vi "Create Engine.vi"(5 "FIFO Debug Flags":refnum<class "Debug Flags FIFO.lvclass">, 7 "fifo/queue depths (10)":u32=10, 8 "error in (no error)":errorcluster, 10 "error size (512 B)":T1=enum."512-byte", 11 "Interface type":refnum<class "Engine Interface.lvclass">) -> (0 "error out":errorcluster, 3 "Interface":refnum<class "Engine Interface.lvclass">)   [LabVIEW 2017, in "Data Sharing Framework Engine.lvlib" / "Engine Interface.lvclass"]
uses:
  Engine Interface.lvclass
  Error Queue Sizes.ctl
  Debug/Debug Flags FIFO/Debug Flags FIFO.lvclass
  Engine Interface.lvclass/Engine Interface.ctl
  Create 16B RT FIFO.vi
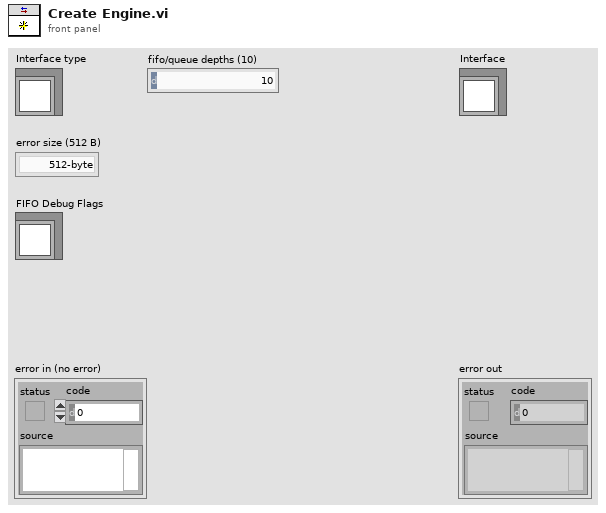
[diagram p1: front panel]
types:
  T1 = typedef "Data Sharing Framework Engine.lvlib/Engine Interface.lvclass/Error Queue Sizes.ctl" = enum16{"256-byte", "512-byte", "1024-byte"}
  T2 = typedef "Data Sharing Framework Engine.lvlib/Engine Interface.lvclass/16B RT FIFO Reference.ctl" = refnum<k33>
  T3 = typedef "Data Sharing Framework Engine.lvlib/Engine Interface.lvclass/Error Queue Ref.ctl" = refnum<queue>
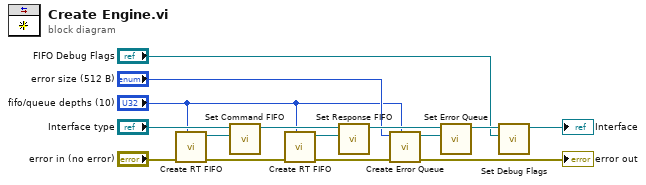
[diagram p0: block diagram]
diagram:
  n1 = call-poly "Create RT FIFO.vi"("size (10)"="fifo/queue depths (10)", "error in (no error)"="error in (no error)") -> ("error out"=w10:errorcluster, "RT FIFO"=w14:T2)  [unwired: 8 in]
  n2 = call "Set Command FIFO.vi"("Command FIFO"=w14, "Interface in"="Interface type") -> ("Interface out"=w11:refnum<class "Engine Interface.lvclass">)  [unwired: 9 in]
  n3 = call-poly "Create RT FIFO.vi"("size (10)"="fifo/queue depths (10)", "error in (no error)"=w10) -> ("error out"=w8:errorcluster, "RT FIFO"=w13:T2)  [unwired: 8 in]
  n4 = call "Set Response FIFO.vi"("Response FIFO"=w13, "Interface in"=w11) -> ("Interface out"=w9:refnum<class "Engine Interface.lvclass">)  [unwired: 9 in]
  n5 = call "Create Error Queue.vi"("max queue size (10)"="fifo/queue depths (10)", "error in (no error)"=w8, "error size"="error size (512 B)") -> ("error out"=→"error out":errorcluster, "Error Queue"=w7:T3)  [unwired: 7 in]
  n6 = call "Set Error Queue.vi"("Error Queue"=w7, "Interface in"=w9) -> ("Interface out"=w4:refnum<class "Engine Interface.lvclass">)  [unwired: 9 in]
  n7 = call "Set Debug Flags.vi"("FIFO Debug Flags"="FIFO Debug Flags", "Interface in"=w4) -> ("Interface out"=→"Interface":refnum<class "Engine Interface.lvclass">)  [unwired: 9 in]
